vi "Deactivate-all-motors.vi"(8 "error in (no error)":errorcluster, 11 "Available motors in":refnum<class "Motor-assembly.lvclass">) -> (0 "error out":errorcluster, 3 "Available motors out":refnum<class "Motor-assembly.lvclass">)   [LabVIEW 2013, in "PowderDeposition.lvlib" / "Motor-assembly.lvclass"]
doc: "Use this template to build a VI to use as a subVI."
uses:
  Motor-assembly.lvclass
  Motor/Motor.lvclass
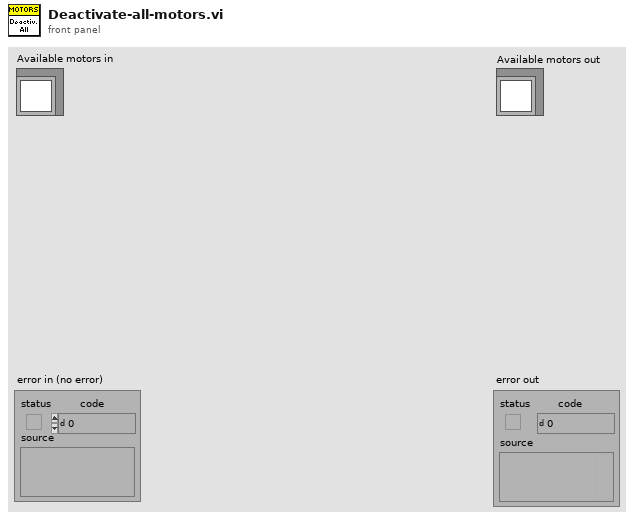
[diagram p1: front panel]
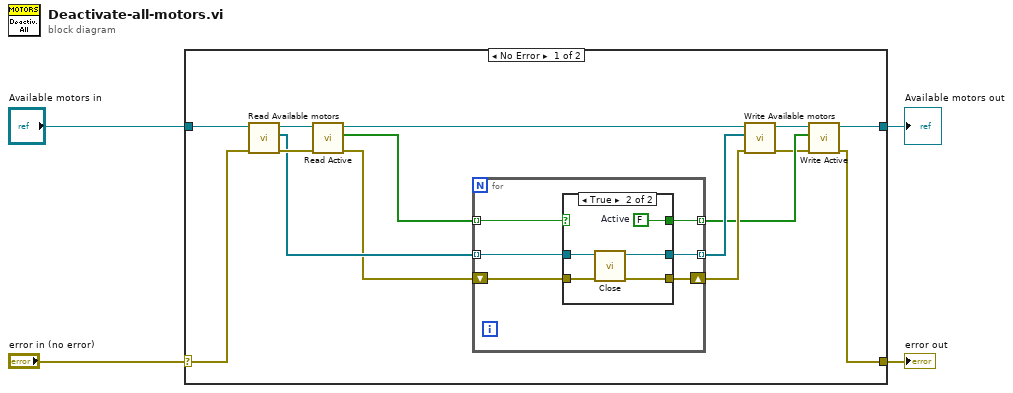
[diagram p0: block diagram]
diagram:
  n1 = case shown="No Error" "error in (no error)" {
    selector: "error in (no error)" -> [w19 w35]
    tunnel: [w7 w35] -> w3
    tunnel: "Available motors in" -> [w6 w34]
    tunnel: [w5 w34] -> w1
    frame No Error {
      n2 = call-dynamic "Read Available motors.vi"("error in (no error)"=w19, "Available motors in"=w6) -> ("error out"=w17:errorcluster, "Available motors"=w15:refnum<class "Motor.lvclass">[], "Available motors out"=w18:refnum<class "Motor-assembly.lvclass">)  [unwired: 7 in]
      n3 = call-dynamic "Read Active.vi"("error in (no error)"=w17, "Available motors in"=w18) -> ("error out"=w14:errorcluster, "Active?"=w16:bool[], "Available motors out"=w11:refnum<class "Motor-assembly.lvclass">)  [unwired: 7 in]
      n4 = for {
        tunnel: w16 -> [w20] mode=indexing
        tunnel: w15 -> [w25] mode=indexing
        tunnel: [w24] -> w12 mode=indexing
        shift-right: [w22] -> w13
        shift-left: w14 -> [w23]
        tunnel: [w21] -> w10 mode=indexing
        n5 = case shown="True" w20 {
          selector: w20 -> [w26 _]
          tunnel: w25 -> [w28 w33]
          tunnel: [w28 w32] -> w24
          tunnel: w23 -> [w27 w31]
          tunnel: [w27 w30] -> w22
          tunnel: [w26 w29] -> w21
          frame False {
          }
          frame True {
            w29 = FALSE  # Active
            n6 = call-dynamic "Close.vi"("error in (no error)"=w31, "Motor in"=w33) -> ("error out"=w30:errorcluster, "Motor out"=w32:refnum<class "Motor.lvclass">)  [unwired: 8 in]
          }
        }
      }
      n7 = call-dynamic "Write Available motors.vi"("error in (no error)"=w13, "Available motors"=w12, "Available motors in"=w11) -> ("error out"=w8:errorcluster, "Available motors out"=w9:refnum<class "Motor-assembly.lvclass">)  [unwired: 7 in]
      n8 = call-dynamic "Write Active.vi"("error in (no error)"=w8, "Active?"=w10, "Available motors in"=w9) -> ("error out"=w7:errorcluster, "Available motors out"=w5:refnum<class "Motor-assembly.lvclass">)  [unwired: 7 in]
    }
    frame Error {
    }
  }
  "error out" <- w3
  "Available motors out" <- w1
